vi "Set Timekeeper CLK10 Input.vi"(5 "Timekeeper":string, 7 "Timekeeper type":T1, 8 "error in (no error)":errorcluster, 10 "Enabled?":bool, 11 "timekeeper in":refnum<k15>) -> (0 "error out":errorcluster, 3 "timekeeper out":refnum<k15>)   [LabVIEW 2018, in "Chassis TimeSync Engine.lvlib"]
uses:
  Chassis TimeSync Engine.lvlib
  timekeeper type.ctl
  Timekeeper Route Pin.ctl
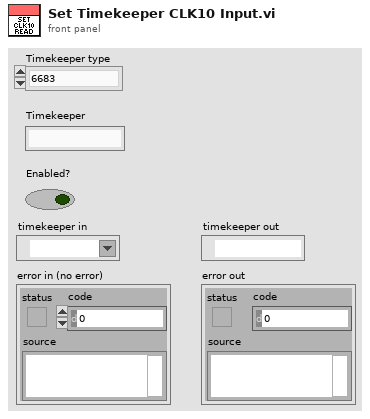
[diagram p1: front panel]
types:
  T1 = typedef "Chassis TimeSync Engine.lvlib/timekeeper type.ctl" = enum16{"6683", "6683H", "6682", "6682H", "non-timekeeper", "timekeeper"}
  T2 = typedef "Chassis TimeSync Engine.lvlib/Timekeeper Route Pin.ctl" = enum16{"TTL0", "PFI0", "PFI1", "PFI2", "PXI_Clk10", "PXI_Clk10_In", "BoardClk", "ClkOut", "Oscillator"}
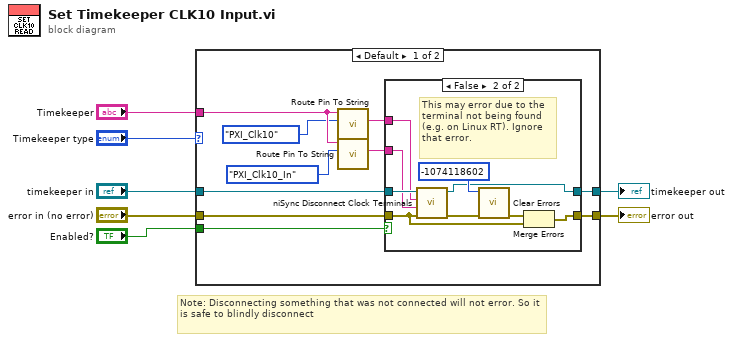
[diagram p0: block diagram]
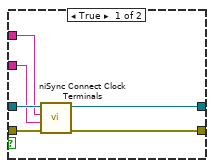
[diagram p2: hidden frame]
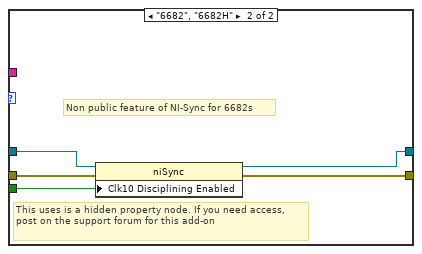
[diagram p3: hidden frame]
diagram:
  # "Note: Disconnecting something that was not connected will not error. So it is safe to blindly disconnect"
  n1 = case shown="Default" "Timekeeper type" {
    tunnel: [w15 w37] -> w7
    tunnel: "timekeeper in" -> [w14 w36]
    tunnel: [w16 w35] -> w5
    tunnel: "error in (no error)" -> [w13 w34]
    tunnel: "Enabled?" -> [w17 w33]
    tunnel: "Timekeeper" -> [w12 _]
    frame Default {
      n2 = call "Route Pin To String.vi"("Pin"=Timekeeper_Route_Pin."PXI_Clk10", "Module"=w12) -> ("String"=w10:string)  [unwired: 9 in]
      n3 = call "Route Pin To String.vi"("Pin"=Timekeeper_Route_Pin."PXI_Clk10_In", "Module"=w12) -> ("String"=w9:string)  [unwired: 9 in]
      n4 = case shown="False" w17 {
        tunnel: [w23 w25] -> w16
        tunnel: [w22 w24] -> w15
        tunnel: w14 -> [w21 w32]
        tunnel: w13 -> [w20 w28]
        tunnel: w10 -> [w19 w31]
        tunnel: w9 -> [w18 w30]
        frame True {
          n5 = call <instrlib>:"niSync Connect Clock Terminals.vi"("error in (no error)"=w20, "destination terminal"=w18, "source terminal"=w19, "instrument handle"=w21) -> ("error out"=w23:errorcluster, "instrument handle out"=w22:refnum<k15>)  [unwired: 6 in]
        }
        frame False {
          # "This may error due to the\nterminal not being found\n(e.g. on Linux RT). Ignore\nthat error."
          n6 = call <instrlib>:"niSync Disconnect Clock Terminals.vi"("error in (no error)"=w28, "destination terminal"=w30, "source terminal"=w31, "instrument handle"=w32) -> ("error out"=w27:errorcluster, "instrument handle out"=w24:refnum<k15>)  [unwired: 6 in]
          n7 = call <vilib>:"Clear Errors.vi"("error in (no error)"=w27, "specific error code to clear (0: all)"=-1074118602) -> ("error out"=w26:errorcluster)  [unwired: 4 in, 1 out]
          n8 = Merge Errors(w26, w28) -> (w25:errorcluster)
        }
      }
    }
    frame "6682", "6682H" {
      # "This uses is a hidden property node. If you need access, post on the support forum for this add-on"
      # "Non public feature of NI-Sync for 6682s"
      n9 = property class="niSync"(reference=w36, error in=w34, "Clk10 Disciplining Enabled"=w33) -> (reference out=w37:refnum<k15>, error out=w35:errorcluster)
    }
  }
  "timekeeper out" <- w7
  "error out" <- w5
